vi "PositionGridCreator.vi"(3 "invert?":bool, 5 "Select order":u16(ring)=1 items=["X->Z->Y"=6, "Y->Z->X"=5, "Z->X->Y"=3, "Y->X->Z"=2, "Z->Y->X"=4, "X->Y->Z"=1], 6 "ScanCoords [mm]":T1) -> (0 "Array of positions":dbl[][](array[numeric]), 1 "Sizes":cluster{i32, i32, i32}, 2 "total number of steps":i32)   [LabVIEW 2015]
panel:
  out "Numeric":i32
  out "Z Array":dbl[](array[numeric])
  out "Y Array":dbl[](array[numeric])
  out "X Array":dbl[](array[numeric])
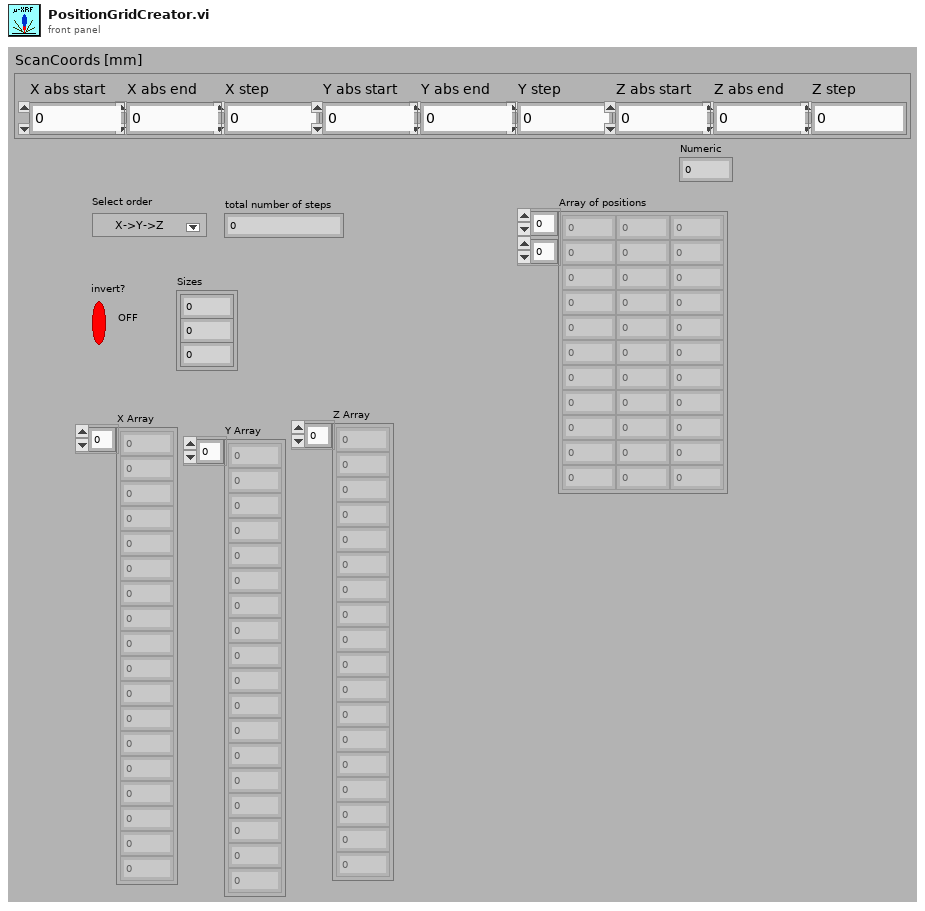
[diagram p1: front panel]
types:
  T1 = cluster{"X abs start":dbl, "X abs end":dbl, "Y abs start":dbl, "Y abs end":dbl, "Z abs start":dbl, "Z abs end":dbl, "X step":dbl, "Y step":dbl, "Z step":dbl}
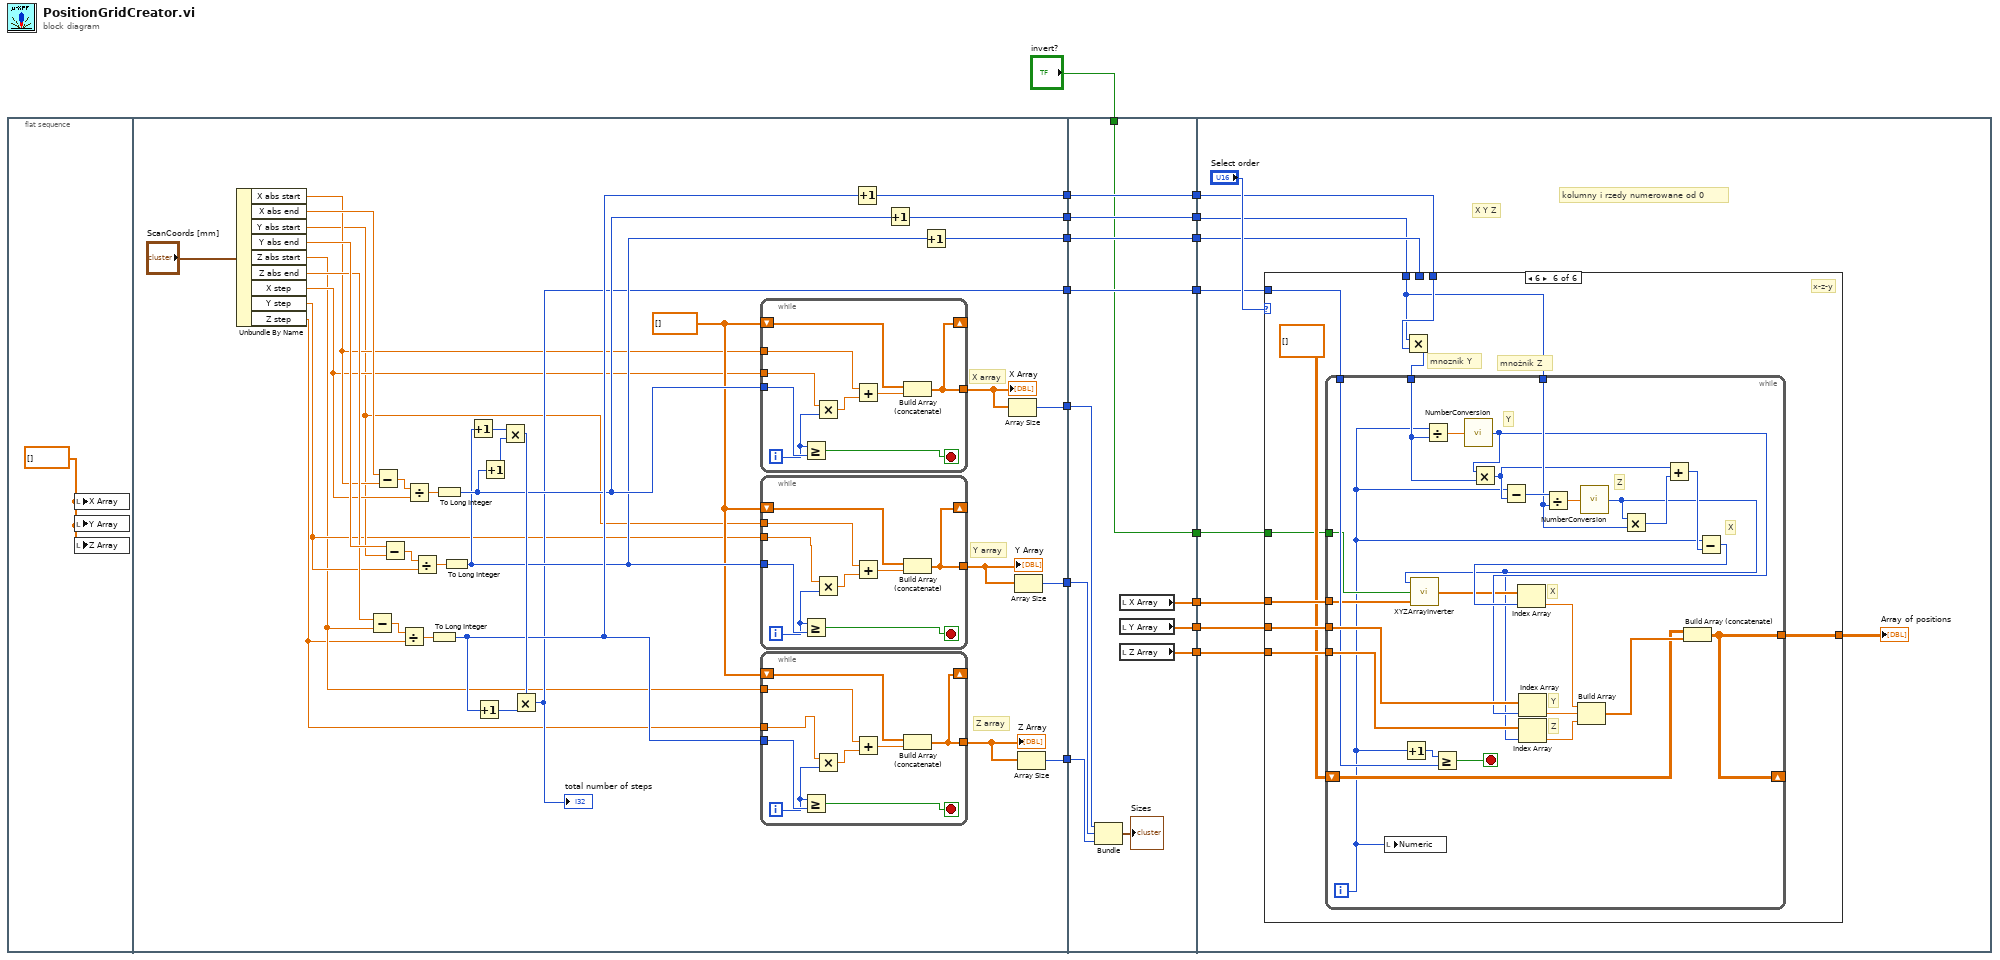
[diagram p0: block diagram]
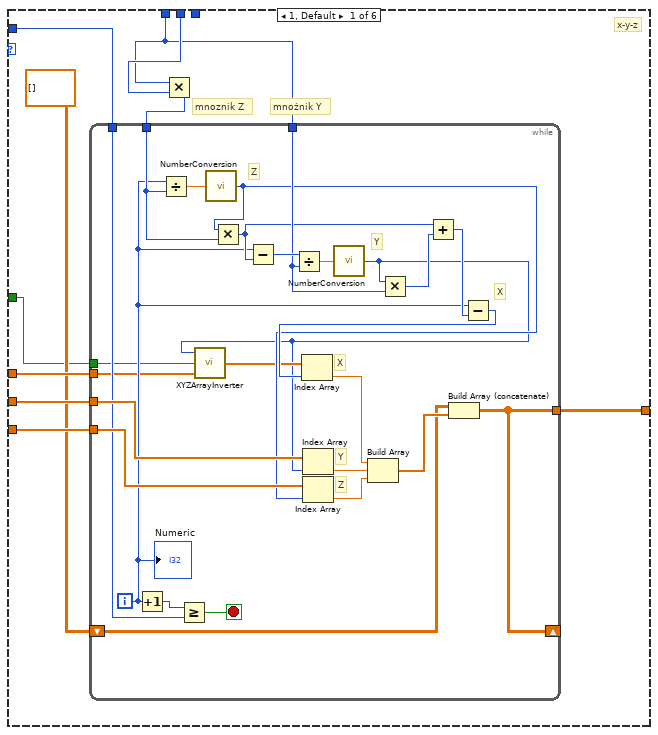
[diagram p2: hidden frame]
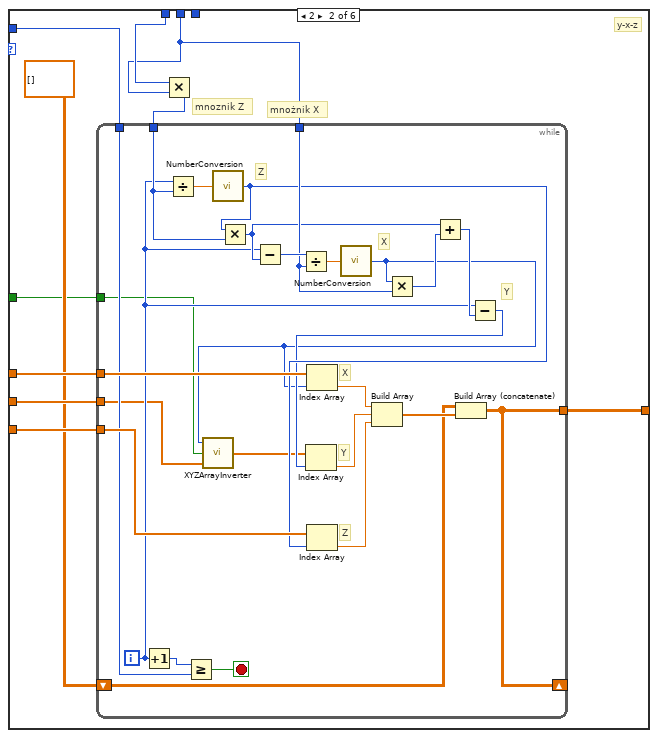
[diagram p3: hidden frame]
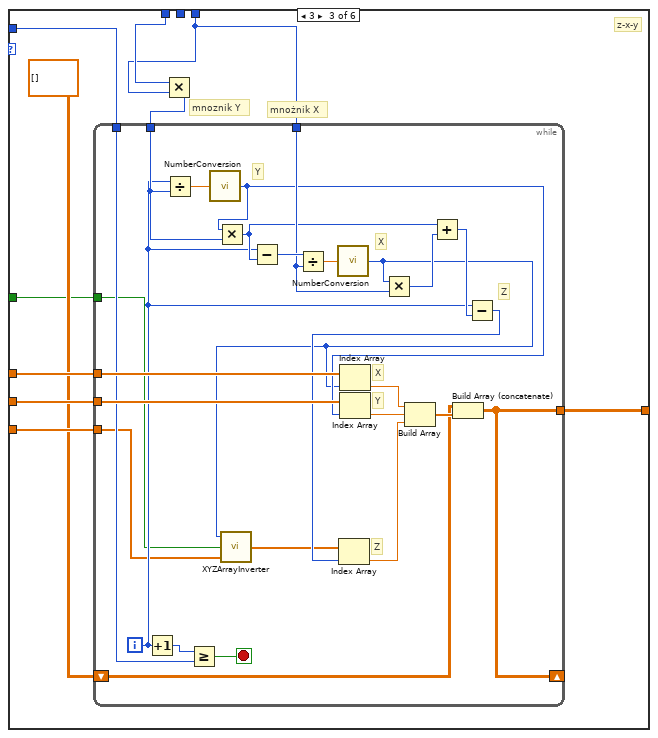
[diagram p4: hidden frame]
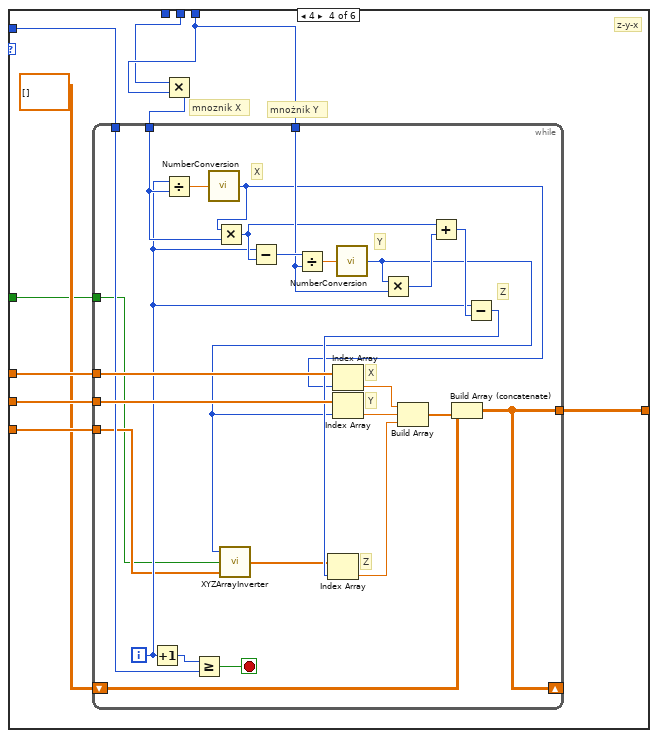
[diagram p5: hidden frame]
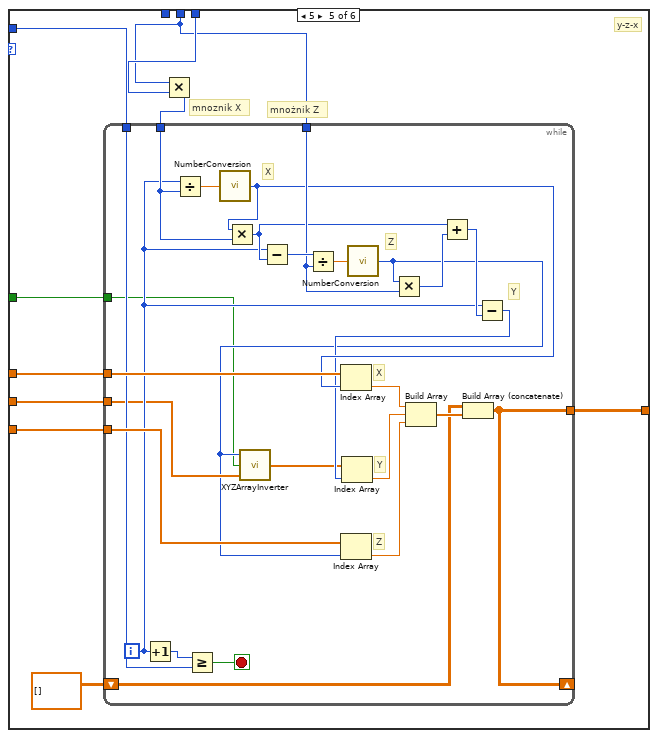
[diagram p6: hidden frame]
diagram:
  n1 = flat-sequence {
    tunnel: [w38] -> w16
    tunnel: [w37] -> w15
    tunnel: [w36] -> w14
    tunnel: [w28] -> w13
    tunnel: [w31] -> w3
    tunnel: [w30] -> w2
    tunnel: [w29] -> w1
    tunnel: w16 -> [w90]
    tunnel: [w90] -> w12
    tunnel: w15 -> [w89]
    tunnel: [w89] -> w11
    tunnel: w14 -> [w88]
    tunnel: [w88] -> w10
    tunnel: w13 -> [w87]
    tunnel: [w87] -> w9
    tunnel: [w86] -> w8
    tunnel: [w85] -> w7
    tunnel: [w84] -> w6
    tunnel: "invert?" -> [w83]
    tunnel: [w83] -> w5
    tunnel: w3 -> [w82]
    tunnel: w2 -> [w81]
    tunnel: w1 -> [w80]
    tunnel: w12 -> [w99]
    tunnel: w11 -> [w98]
    tunnel: w10 -> [w96]
    tunnel: w9 -> [w97]
    tunnel: w8 -> [w93]
    tunnel: w7 -> [w94]
    tunnel: w6 -> [w95]
    tunnel: w5 -> [w91]
    frame #0 {
      w17 = dbl[] [] ("initialized array")
      n2 = local write "X Array"(w17) -> ()
      n3 = local write "Y Array"(w17) -> ()
      n4 = local write "Z Array"(w17) -> ()
    }
    frame #1 {
      w35 = dbl[] []
      # "Z array"
      # "Y array"
      # "X array"
      n5 = Unbundle By Name("ScanCoords [mm]") -> ("X abs start"=w23:dbl, "X abs end"=w26:dbl, "Y abs start"=w21:dbl, "Y abs end"=w25:dbl, "Z abs start"=w19:dbl, "Z abs end"=w24:dbl, "X step"=w22:dbl, "Y step"=w20:dbl, "Z step"=w18:dbl)
      n6 = Subtract(x=w24, y=w19) -> (x-y=w46:dbl)
      n7 = Subtract(x=w26, y=w23) -> (x-y=w42:dbl)
      n8 = Subtract(x=w25, y=w21) -> (x-y=w44:dbl)
      n9 = Divide(x=w46, y=w18) -> (x/y=w47:dbl)
      n10 = Divide(x=w42, y=w22) -> (x/y=w43:dbl)
      n11 = Divide(x=w44, y=w20) -> (x/y=w45:dbl)
      n12 = To Long Integer(number=w47) -> (32bit integer=w41:i32)
      n13 = To Long Integer(number=w43) -> (32bit integer=w40:i32)
      n14 = To Long Integer(number=w45) -> (32bit integer=w39:i32)
      n15 = Increment(x=w39) -> (x+1=w49:i32)
      n16 = Increment(x=w41) -> (x+1=w51:i32)
      n17 = Increment(x=w40) -> (x+1=w50:i32)
      n18 = Multiply(x=w49, y=w50) -> (x*y=w48:i32)
      n19 = Multiply(x=w48, y=w51) -> (x*y=w28:i32)
      "total number of steps" <- w28
      n20 = while {
        tunnel: w40 -> [w78]
        tunnel: [w72] -> w34
        shift-right: [w72] -> _
        shift-left: w35 -> [w73]
        tunnel: w23 -> [w71]
        tunnel: w22 -> [w70]
        i -> [w76]
        stop <- w77 stop-if-true
        n21 = Greater Or Equal?(x=w76, y=w78) -> (x >= y?=w77:bool)
        n22 = Multiply(x=w70, y=w76) -> (x*y=w75:dbl)
        n23 = Add(x=w71, y=w75) -> (x+y=w74:dbl)
        n24 = Build Array (concatenate)(w73, w74) -> (w72:dbl[])
      }
      "X Array" <- w34
      n25 = while {
        tunnel: w39 -> [w69]
        tunnel: [w64] -> w33
        shift-right: [w64] -> _
        shift-left: w35 -> [w63]
        tunnel: w21 -> [w62]
        tunnel: w20 -> [w61]
        i -> [w67]
        stop <- w68 stop-if-true
        n26 = Greater Or Equal?(x=w67, y=w69) -> (x >= y?=w68:bool)
        n27 = Multiply(x=w61, y=w67) -> (x*y=w66:dbl)
        n28 = Add(x=w62, y=w66) -> (x+y=w65:dbl)
        n29 = Build Array (concatenate)(w63, w65) -> (w64:dbl[])
      }
      "Y Array" <- w33
      n30 = while {
        tunnel: w41 -> [w60]
        tunnel: [w55] -> w32
        shift-right: [w55] -> _
        shift-left: w35 -> [w54]
        tunnel: w19 -> [w53]
        tunnel: w18 -> [w52]
        i -> [w58]
        stop <- w59 stop-if-true
        n31 = Greater Or Equal?(x=w58, y=w60) -> (x >= y?=w59:bool)
        n32 = Multiply(x=w52, y=w58) -> (x*y=w57:dbl)
        n33 = Add(x=w53, y=w57) -> (x+y=w56:dbl)
        n34 = Build Array (concatenate)(w54, w56) -> (w55:dbl[])
      }
      "Z Array" <- w32
      n35 = Increment(x=w41) -> (x+1=w36:i32)
      n36 = Increment(x=w40) -> (x+1=w37:i32)
      n37 = Increment(x=w39) -> (x+1=w38:i32)
      n38 = Array Size(array=w34) -> (size(s)=w31:i32)
      n39 = Array Size(array=w33) -> (size(s)=w30:i32)
      n40 = Array Size(array=w32) -> (size(s)=w29:i32)
    }
    frame #2 {
      n41 = Bundle(w82, w81, w80) -> (→"Sizes":cluster{i32, i32, i32})  [unwired: 1 in]
      n42 = local read "X Array"() -> (w84:dbl[])
      n43 = local read "Y Array"() -> (w85:dbl[])
      n44 = local read "Z Array"() -> (w86:dbl[])
    }
    frame #3 {
      # "X Y Z"
      # "kolumny i rzedy numerowane od 0"
      n45 = case shown="6" "Select order" {
        tunnel: w95 -> [w107 w144 w180 w217 w253 w289]
        tunnel: w94 -> [w106 w143 w179 w216 w252 w288]
        tunnel: w93 -> [w105 w142 w178 w215 w251 w287]
        tunnel: w97 -> [w104 w141 w177 w214 w250 w286]
        tunnel: w98 -> [w108 w145 w181 _ _ w283]
        tunnel: w99 -> [w110 w139 _ w211 w247 _]
        tunnel: w96 -> [_ _ w175 w212 w248 w284]
        tunnel: [w103 w140 w176 w213 w249 w285] -> w92
        tunnel: w91 -> [w101 w137 w173 w209 w245 w281]
        frame 1, Default {
          # "x-y-z"
          # "mnożnik Y"
          # "mnoznik Z"
          n46 = Multiply(x=w108, y=w110) -> (x*y=w109:i32)
          n47 = while {
            tunnel: w109 -> [w135]
            tunnel: w108 -> [w132]
            tunnel: w107 -> [w114]
            tunnel: w106 -> [w127]
            tunnel: w105 -> [w126]
            tunnel: w104 -> [w124]
            tunnel: [w115] -> w103
            shift-right: [w115] -> _
            shift-left: dbl[][] [] -> [w116]
            tunnel: w101 -> [w111]
            i -> [w118]
            stop <- w123 stop-if-true
            # "Z"
            # "Y"
            # "X"
            # "X"
            # "Y"
            # "Z"
            n48 = Increment(x=w118) -> (x+1=w117:i32)
            n49 = Divide(x=w118, y=w135) -> (x/y=w136:dbl)
            n50 = Greater Or Equal?(x=w117, y=w124) -> (x >= y?=w123:bool)
            n51 = call "NumberConversion.vi"("Numeric"=w136) -> ("number"=w125:i32)
            n52 = Multiply(x=w125, y=w135) -> (x*y=w131:i32)
            n53 = Subtract(x=w118, y=w131) -> (x-y=w134:i32)
            n54 = Divide(x=w134, y=w132) -> (x/y=w133:dbl)
            n55 = Index Array(array=w126, index=w125) -> (element=w121:dbl)
            n56 = call "NumberConversion.vi"("Numeric"=w133) -> ("number"=w112:i32)
            n57 = call "XYZArrayInverter.vi"("input array"=w114, "invert?"=w111, "Number"=w112) -> ("modified array"=w113:dbl[])
            n58 = Index Array(array=w127, index=w112) -> (element=w120:dbl)
            n59 = Multiply(x=w112, y=w132) -> (x*y=w130:i32)
            n60 = Add(x=w131, y=w130) -> (x+y=w129:i32)
            n61 = Subtract(x=w118, y=w129) -> (x-y=w128:i32)
            n62 = Index Array(array=w113, index=w128) -> (element=w122:dbl)
            n63 = Build Array(w122, w120, w121) -> (w119:dbl[])
            n64 = Build Array (concatenate)(w116, w119) -> (w115:dbl[][])
            "Numeric" <- w118
          }
        }
        frame 2 {
          # "y-x-z"
          # "mnożnik X"
          # "mnoznik Z"
          n65 = Multiply(x=w145, y=w139) -> (x*y=w146:i32)
          n66 = while {
            tunnel: w146 -> [w171]
            tunnel: w139 -> [w168]
            tunnel: w144 -> [w164]
            tunnel: w143 -> [w150]
            tunnel: w142 -> [w163]
            tunnel: w141 -> [w161]
            tunnel: [w151] -> w140
            shift-right: [w151] -> _
            shift-left: dbl[][] [] -> [w152]
            tunnel: w137 -> [w147]
            i -> [w155]
            stop <- w160 stop-if-true
            # "Z"
            # "Y"
            # "X"
            # "Y"
            # "X"
            # "Z"
            n67 = Increment(x=w155) -> (x+1=w154:i32)
            n68 = Divide(x=w155, y=w171) -> (x/y=w172:dbl)
            n69 = Greater Or Equal?(x=w154, y=w161) -> (x >= y?=w160:bool)
            n70 = call "NumberConversion.vi"("Numeric"=w172) -> ("number"=w162:i32)
            n71 = Multiply(x=w162, y=w171) -> (x*y=w167:i32)
            n72 = Subtract(x=w155, y=w167) -> (x-y=w170:i32)
            n73 = Divide(x=w170, y=w168) -> (x/y=w169:dbl)
            n74 = Index Array(array=w163, index=w162) -> (element=w158:dbl)
            n75 = call "NumberConversion.vi"("Numeric"=w169) -> ("number"=w148:i32)
            n76 = call "XYZArrayInverter.vi"("input array"=w150, "invert?"=w147, "Number"=w148) -> ("modified array"=w149:dbl[])
            n77 = Index Array(array=w164, index=w148) -> (element=w159:dbl)
            n78 = Multiply(x=w148, y=w168) -> (x*y=w166:i32)
            n79 = Add(x=w167, y=w166) -> (x+y=w165:i32)
            n80 = Subtract(x=w155, y=w165) -> (x-y=w153:i32)
            n81 = Index Array(array=w149, index=w153) -> (element=w157:dbl)
            n82 = Build Array(w159, w157, w158) -> (w156:dbl[])
            n83 = Build Array (concatenate)(w152, w156) -> (w151:dbl[][])
          }
        }
        frame 3 {
          # "z-x-y"
          # "mnożnik X"
          # "mnoznik Y"
          n84 = Multiply(x=w181, y=w175) -> (x*y=w182:i32)
          n85 = while {
            tunnel: w182 -> [w207]
            tunnel: w175 -> [w204]
            tunnel: w180 -> [w200]
            tunnel: w179 -> [w199]
            tunnel: w178 -> [w186]
            tunnel: w177 -> [w198]
            tunnel: [w187] -> w176
            shift-right: [w187] -> _
            shift-left: dbl[][] [] -> [w188]
            tunnel: w173 -> [w183]
            i -> [w192]
            stop <- w197 stop-if-true
            # "Z"
            # "Y"
            # "X"
            # "Z"
            # "X"
            # "Y"
            n86 = Increment(x=w192) -> (x+1=w191:i32)
            n87 = Divide(x=w192, y=w207) -> (x/y=w208:dbl)
            n88 = Greater Or Equal?(x=w191, y=w198) -> (x >= y?=w197:bool)
            n89 = call "NumberConversion.vi"("Numeric"=w208) -> ("number"=w189:i32)
            n90 = Multiply(x=w189, y=w207) -> (x*y=w203:i32)
            n91 = Subtract(x=w192, y=w203) -> (x-y=w206:i32)
            n92 = Divide(x=w206, y=w204) -> (x/y=w205:dbl)
            n93 = call "NumberConversion.vi"("Numeric"=w205) -> ("number"=w184:i32)
            n94 = call "XYZArrayInverter.vi"("input array"=w186, "invert?"=w183, "Number"=w184) -> ("modified array"=w185:dbl[])
            n95 = Index Array(array=w200, index=w184) -> (element=w196:dbl)
            n96 = Index Array(array=w199, index=w189) -> (element=w194:dbl)
            n97 = Multiply(x=w184, y=w204) -> (x*y=w202:i32)
            n98 = Add(x=w203, y=w202) -> (x+y=w201:i32)
            n99 = Subtract(x=w192, y=w201) -> (x-y=w190:i32)
            n100 = Index Array(array=w185, index=w190) -> (element=w195:dbl)
            n101 = Build Array(w196, w194, w195) -> (w193:dbl[])
            n102 = Build Array (concatenate)(w188, w193) -> (w187:dbl[][])
          }
        }
        frame 4 {
          # "z-y-x"
          # "mnożnik Y"
          # "mnoznik X"
          n103 = Multiply(x=w211, y=w212) -> (x*y=w218:i32)
          n104 = while {
            tunnel: w218 -> [w243]
            tunnel: w212 -> [w240]
            tunnel: w217 -> [w236]
            tunnel: w216 -> [w235]
            tunnel: w215 -> [w222]
            tunnel: w214 -> [w234]
            tunnel: [w224] -> w213
            shift-right: [w224] -> _
            shift-left: dbl[][] [] -> [w223]
            tunnel: w209 -> [w219]
            i -> [w228]
            stop <- w233 stop-if-true
            # "Z"
            # "Y"
            # "X"
            # "Z"
            # "Y"
            # "X"
            n105 = Increment(x=w228) -> (x+1=w227:i32)
            n106 = Divide(x=w228, y=w243) -> (x/y=w244:dbl)
            n107 = Greater Or Equal?(x=w227, y=w234) -> (x >= y?=w233:bool)
            n108 = call "NumberConversion.vi"("Numeric"=w244) -> ("number"=w225:i32)
            n109 = Multiply(x=w225, y=w243) -> (x*y=w239:i32)
            n110 = Subtract(x=w228, y=w239) -> (x-y=w242:i32)
            n111 = Divide(x=w242, y=w240) -> (x/y=w241:dbl)
            n112 = Index Array(array=w236, index=w225) -> (element=w232:dbl)
            n113 = call "NumberConversion.vi"("Numeric"=w241) -> ("number"=w220:i32)
            n114 = call "XYZArrayInverter.vi"("input array"=w222, "invert?"=w219, "Number"=w220) -> ("modified array"=w221:dbl[])
            n115 = Index Array(array=w235, index=w220) -> (element=w230:dbl)
            n116 = Multiply(x=w220, y=w240) -> (x*y=w238:i32)
            n117 = Add(x=w239, y=w238) -> (x+y=w237:i32)
            n118 = Subtract(x=w228, y=w237) -> (x-y=w226:i32)
            n119 = Index Array(array=w221, index=w226) -> (element=w231:dbl)
            n120 = Build Array(w232, w230, w231) -> (w229:dbl[])
            n121 = Build Array (concatenate)(w223, w229) -> (w224:dbl[][])
          }
        }
        frame 5 {
          # "y-z-x"
          # "mnożnik Z"
          # "mnoznik X"
          n122 = Multiply(x=w247, y=w248) -> (x*y=w254:i32)
          n123 = while {
            tunnel: w254 -> [w279]
            tunnel: w247 -> [w276]
            tunnel: w253 -> [w272]
            tunnel: w252 -> [w257]
            tunnel: w251 -> [w271]
            tunnel: w250 -> [w270]
            tunnel: [w259] -> w249
            shift-right: [w259] -> _
            shift-left: dbl[][] [] -> [w260]
            tunnel: w245 -> [w255]
            i -> [w264]
            stop <- w269 stop-if-true
            # "Z"
            # "Y"
            # "X"
            # "Y"
            # "Z"
            # "X"
            n124 = Increment(x=w264) -> (x+1=w263:i32)
            n125 = Divide(x=w264, y=w279) -> (x/y=w280:dbl)
            n126 = Greater Or Equal?(x=w263, y=w270) -> (x >= y?=w269:bool)
            n127 = call "NumberConversion.vi"("Numeric"=w280) -> ("number"=w262:i32)
            n128 = Multiply(x=w262, y=w279) -> (x*y=w275:i32)
            n129 = Subtract(x=w264, y=w275) -> (x-y=w278:i32)
            n130 = Divide(x=w278, y=w276) -> (x/y=w277:dbl)
            n131 = Index Array(array=w272, index=w262) -> (element=w268:dbl)
            n132 = call "NumberConversion.vi"("Numeric"=w277) -> ("number"=w256:i32)
            n133 = call "XYZArrayInverter.vi"("input array"=w257, "invert?"=w255, "Number"=w256) -> ("modified array"=w258:dbl[])
            n134 = Index Array(array=w271, index=w256) -> (element=w267:dbl)
            n135 = Multiply(x=w256, y=w276) -> (x*y=w274:i32)
            n136 = Add(x=w275, y=w274) -> (x+y=w273:i32)
            n137 = Subtract(x=w264, y=w273) -> (x-y=w261:i32)
            n138 = Index Array(array=w258, index=w261) -> (element=w266:dbl)
            n139 = Build Array(w268, w266, w267) -> (w265:dbl[])
            n140 = Build Array (concatenate)(w260, w265) -> (w259:dbl[][])
          }
        }
        frame 6 {
          # "x-z-y"
          # "mnożnik Z"
          # "mnoznik Y"
          n141 = Multiply(x=w283, y=w284) -> (x*y=w290:i32)
          n142 = while {
            tunnel: w290 -> [w315]
            tunnel: w283 -> [w312]
            tunnel: w289 -> [w295]
            tunnel: w288 -> [w308]
            tunnel: w287 -> [w307]
            tunnel: w286 -> [w306]
            tunnel: [w297] -> w285
            shift-right: [w297] -> _
            shift-left: dbl[][] [] -> [w296]
            tunnel: w281 -> [w292]
            i -> [w291]
            stop <- w305 stop-if-true
            # "Z"
            # "Y"
            # "X"
            # "X"
            # "Z"
            # "Y"
            n143 = local write "Numeric"(w291) -> ()
            n144 = Increment(x=w291) -> (x+1=w300:i32)
            n145 = Divide(x=w291, y=w315) -> (x/y=w316:dbl)
            n146 = Greater Or Equal?(x=w300, y=w306) -> (x >= y?=w305:bool)
            n147 = call "NumberConversion.vi"("Numeric"=w316) -> ("number"=w298:i32)
            n148 = Multiply(x=w298, y=w315) -> (x*y=w311:i32)
            n149 = Subtract(x=w291, y=w311) -> (x-y=w314:i32)
            n150 = Index Array(array=w308, index=w298) -> (element=w302:dbl)
            n151 = Divide(x=w314, y=w312) -> (x/y=w313:dbl)
            n152 = call "NumberConversion.vi"("Numeric"=w313) -> ("number"=w293:i32)
            n153 = call "XYZArrayInverter.vi"("input array"=w295, "invert?"=w292, "Number"=w293) -> ("modified array"=w294:dbl[])
            n154 = Index Array(array=w307, index=w293) -> (element=w303:dbl)
            n155 = Multiply(x=w293, y=w312) -> (x*y=w310:i32)
            n156 = Add(x=w311, y=w310) -> (x+y=w309:i32)
            n157 = Subtract(x=w291, y=w309) -> (x-y=w299:i32)
            n158 = Index Array(array=w294, index=w299) -> (element=w304:dbl)
            n159 = Build Array(w304, w302, w303) -> (w301:dbl[])
            n160 = Build Array (concatenate)(w296, w301) -> (w297:dbl[][])
          }
        }
      }
      "Array of positions" <- w92
    }
  }
